vi "ErrorToString.vi"(9 "Error in":errorcluster, 10 "Appended error index":i32=-1 caption="Appended error index (-1)") -> (1 "Error as string":string)   [LabVIEW 2017, in "GPError.lvlib"]
doc: "Formats the <B>Error in</B> cluster into <B>Error as string</B> following this pattern;\n\n\"[<index>] Error/Warning code <code>, Source: <source>, Time: <timestamp>, <description 1>, <description 2>...<description n>\"\n\nwhere:\n\n<index> is <B>Appended error index</B>.\n<code> is the code field from <B>Error in</B>.\n<source> is the decoded source value from <B>Error in</B> (that's not the same as the source field from <B>Error in</B>).\n<timestamp> is the embedded timestamp from the SetTimestamp function. This field will be omitted if there is no timestamp present.\n<description 1..n> are the calculated description strings from the concrete error in <B>Error in</B>.\n\nIf <B>Appended error index</B> is less than zero the entire \"[<index>] \" part will be omitted from the <B>Error as string</B>.\n\nSteen Schmidt\nGPower\n15/11 2014"
uses:
  GPError.lvlib
panel:
  # "Copyright © 2014\nGPower\nSee enclosed license file for terms and conditions"
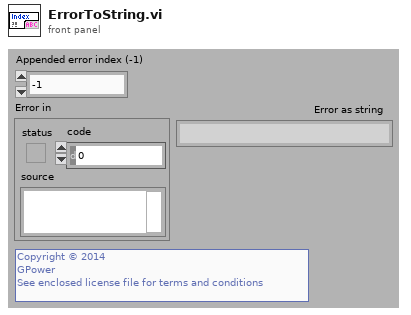
[diagram p1: front panel]
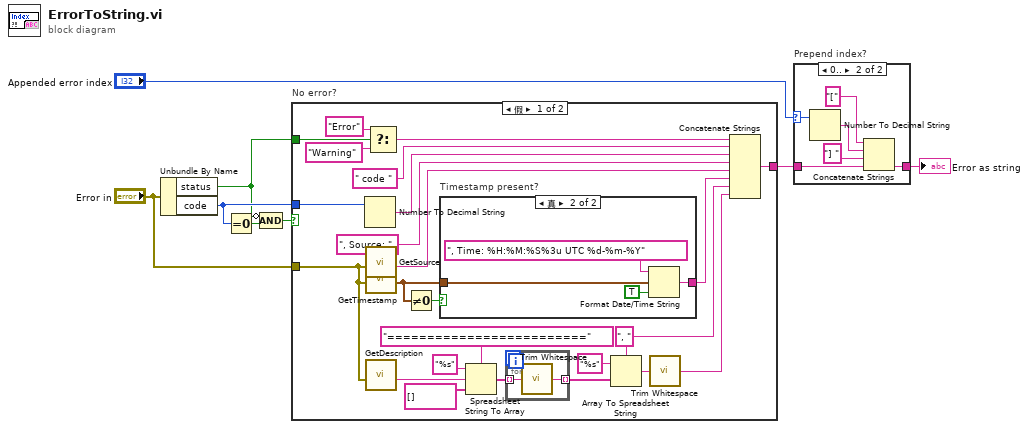
[diagram p0: block diagram]
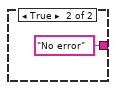
[diagram p3: hidden frame]
diagram:
  n1 = Unbundle By Name("Error in") -> ("status"=w2:bool, "code"=w4:i32)
  n2 = Equal To 0?(x=w4) -> (x = 0?=w3:bool)
  n3 = Compound Arithmetic op=AND(invert w2, w3) -> (w1:bool)
  n4 = case "No error?" shown="假" w1 {
    tunnel: w2 -> [w32 _]
    tunnel: w4 -> [w15 _]
    tunnel: "Error in" -> [w14 _]
    tunnel: [w16 "No error"] -> w6
    frame False {
      w11 = ", " ("delimiter (Tab)")
      n5 = Number To Decimal String(number=w15) -> (decimal integer string=w27:string)  [unwired: 1 in]
      n6 = call "GetSource.vi"("Error in"=w14) -> ("Source"=w25:string)  [unwired: 10 in]
      n7 = call "GetTimestamp.vi"("Error in"=w14) -> ("Timestamp"=w10:timestamp)  [unwired: 10 in]
      n8 = call "GetDescription.vi"("Error in"=w14) -> ("Description"=w20:string)  [unwired: 10 in]
      n9 = Select(t="Error", s=w32, f="Warning") -> (s? t:f=w29:string)
      n10 = Not Equal To 0?(x=w10) -> (x != 0?=w13:bool)
      n11 = case "Timestamp present?" shown="真" w13 {
        tunnel: w10 -> [_ w34]
        tunnel: [_ w33] -> w9
        frame False {
        }
        frame True {
          n12 = Format Date/Time String(time format string (%c)=", Time: %H:%M:%S%3u UTC %d-%m-%Y", seconds (now)=w34, UTC format=TRUE) -> (date/time string=w33:string)
        }
      }
      n13 = Spreadsheet String To Array(delimiter (Tab)="=========================", format string="%s", spreadsheet string=w20, array type (2D Dbl)=string[] []) -> (array=w22:string[])
      n14 = for {
        tunnel: w22 -> [w38] mode=indexing
        tunnel: [w37] -> w19 mode=indexing
        n15 = call <vilib>:"Trim Whitespace.vi"("string"=w38) -> ("trimmed string"=w37:string)  [unwired: 1 in]
      }
      n16 = Array To Spreadsheet String(delimiter (Tab)=w11, array=w19, 3:"%s" ("format string")) -> (spreadsheet string=w17:string)
      n17 = call <vilib>:"Trim Whitespace.vi"("string"=w17) -> ("trimmed string"=w12:string)  [unwired: 1 in]
      n18 = Concatenate Strings(w29, " code ", w27, ", Source: ", w25, w9, w11, w12) -> (w16:string)
    }
    frame True {
    }
  }
  n19 = case "Prepend index?" shown="0.." "Appended error index" {
    selector: "Appended error index" -> [_ w46]
    tunnel: w6 -> [w40 w45]
    tunnel: [w40 w41] -> w5
    frame ..-1 {
    }
    frame 0.. {
      n20 = Number To Decimal String(number=w46) -> (decimal integer string=w43:string)  [unwired: 1 in]
      n21 = Concatenate Strings("[", w43, "] ", w45) -> (w41:string)
    }
  }
  "Error as string" <- w5
